vi "Stop Core.vi"(10 "final error code":i32, 11 "O3 Frequency Train Actor in":refnum<class "O3 Frequency Train Actor.lvclass">) -> (3 "O3 Frequency Train Actor out":refnum<class "O3 Frequency Train Actor.lvclass">)   [LabVIEW 2014, in "Calibration.lvlib" / "O3 Frequency Train Actor.lvclass"]
doc: "(<B>Filename</B>: Actor Framework.lvlib:Actor.lvclass:Stop Core.vi)\n\nDefines what the actor does before it stops. Use the <B>final error code</B> input to determine whether the actor shut down in response to an error.\n\nBy default, this method does nothing. A descendant class may override it to define behavior, such as shutting down any processes the actor initiated in its override of the Actor Core method."
uses:
  O3 Frequency Train Actor.lvclass
  SuperActor/SuperActor.lvclass
  reusable/Session APIs/Session Log/System Log.lvclass
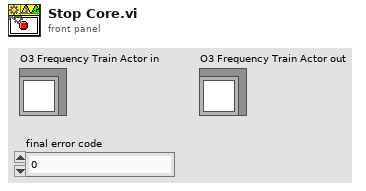
[diagram p1: front panel]
types:
  T1 = typedef "Session - Root.lvclass/Session Handle.ctl" = refnum<data-value>
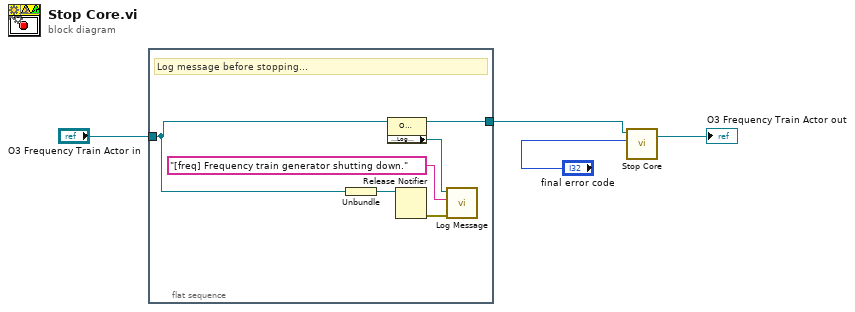
[diagram p0: block diagram]
diagram:
  n1 = flat-sequence {
    tunnel: "O3 Frequency Train Actor in" -> [w9]
    tunnel: [w6] -> w1
    frame #0 {
      # "Log message before stopping..."
      n2 = Unbundle(w9) -> (w10:refnum<notifier>)
      n3 = property class="O3 Frequency Train Actors"(reference=w9) -> (reference out=w6:refnum<class "O3 Frequency Train Actor.lvclass">, "Accessors:Log Session"=w8:T1)  [unwired: 1 in, 1 out]
      n4 = Release Notifier(notifier=w10) -> (error out=w5:errorcluster)  [unwired: 2 in, 2 out]
      n5 = call "Log Message.vi"("error in"=w5, "MSG In"="[freq] Frequency train generator shutting down.", "session in"=w8) -> ()  [unwired: 7 in, 2 out]
    }
  }
  n6 = call-parent "Stop Core.vi"("final error code"="final error code", "Ex Nested in"=w1) -> ("Ex Nested out"=→"O3 Frequency Train Actor out":refnum<class "O3 Frequency Train Actor.lvclass">)  [unwired: 9 in]
